vi "AddObject.vi"(6 "donating?":bool=TRUE, 8 "error in (no error)":errorcluster, 9 "Ancestor":string, 10 "driver":refnum<class "ViPER.lvclass">, 11 "reference in":refnum<class "ViPER.lvclass">) -> (0 "error out":errorcluster, 3 "reference out":refnum<class "ViPER.lvclass">)   [LabVIEW 2022 SP3, in "ViPER.lvlib" / "ViPER.lvclass"]
doc: "### BSD License (http://www.opensource.org/licenses/bsd-license.php) Begin ###\n\nCopyright (c) 2018 Kurt Friday www.medulla.net\n\nAll rights reserved.\n\nRedistribution and use in source and binary forms, with or without\nmodification, are permitted provided that the following conditions are met:\n\n * Redistributions of source code must retain the above copyright\n notice, this list of conditions and the following disclaimer.\n\n * Redistributions in binary form must reproduce the above copyright\n notice, this list of conditions and the following disclaimer in the\n documentation and/or other materials provided with the distribution.\n\n * Neither the name of the <organization> nor the\n names of its contributors may be used to endorse or promote products\n derived from this software without specific prior written permission.\n\nTHIS SOFTWARE IS PROVIDED BY THE COPYRIGHT HOLDERS AND CONTRIBUTORS \"AS IS\" AND\nANY EXPRESS OR IMPLIED WARRANTIES, INCLUDING, BUT NOT LIMITED TO, THE IMPLIED\nWARRANTIES OF MERCHANTABILITY AND FITNESS FOR A PARTICULAR PURPOSE ARE\nDISCLAIMED. IN NO EVENT SHALL <COPYRIGHT HOLDER> BE LIABLE FOR ANY\nDIRECT, INDIRECT, INCIDENTAL, SPECIAL, EXEMPLARY, OR CONSEQUENTIAL DAMAGES\n(INCLUDING, BUT NOT LIMITED TO, PROCUREMENT OF SUBSTITUTE GOODS OR SERVICES;\nLOSS OF USE, DATA, OR PROFITS; OR BUSINESS INTERRUPTION) HOWEVER CAUSED AND\nON ANY THEORY OF LIABILITY, WHETHER IN CONTRACT, STRICT LIABILITY, OR TORT\n(INCLUDING NEGLIGENCE OR OTHERWISE) ARISING IN ANY WAY OUT OF THE USE OF THIS\nSOFTWARE, EVEN IF ADVISED OF THE POSSIBILITY OF SUCH DAMAGE."
uses:
  ViPER.lvclass
  ObjectLayers.ctl
panel:
  # "### BSD License (http://www.opensource.org/licenses/bsd-license.php) Begin ###\n\nCopyright (c) 2018  Kurt Friday www.medulla.net\n\nAll rights reserved.\n\nRedistribution and use in source and binary forms, with or without\nmodification, are permitted provided that the following conditions are met:\n\n    * Redistributions of source code must retain the above copyright\n      notice, this list of conditions and the following disclaimer.\n\n    * Redistributions in binary form must reproduce the above copyright\n      notice, this list of conditions and the following disclaimer in the\n      documentation and/or other materials provided with the distribution.\n\n    * Neither the name of the <organization> nor the\n      names of its contributors may be used to endorse or promote products\n      derived from this software without specific prior written permission.\n\nTHIS SOFTWARE IS PROVIDED BY THE COPYRIGHT HOLDERS AND CONTRIBUTORS \"AS IS\" AND\nANY EXPRESS OR IMPLIED WARRANTIES, INCLUDING, BUT NOT LIMITED TO, THE IMPLIED\nWARRANTIES OF MERCHANTABILITY AND FITNESS FOR A PARTICULAR PURPOSE ARE\nDISCLAIMED. IN NO EVENT SHALL <COPYRIGHT HOLDER> BE LIABLE FOR ANY\nDIRECT, INDIRECT, INCIDENTAL, SPECIAL, EXEMPLARY, OR CONSEQUENTIAL DAMAGES\n(INCLUDING, BUT NOT LIMITED TO, PROCUREMENT OF SUBSTITUTE GOODS OR SERVICES;\nLOSS OF USE, DATA, OR PROFITS; OR BUSINESS INTERRUPTION) HOWEVER CAUSED AND\nON ANY THEORY OF LIABILITY, WHETHER IN CONTRACT, STRICT LIABILITY, OR TORT\n(INCLUDING NEGLIGENCE OR OTHERWISE) ARISING IN ANY WAY OUT OF THE USE OF THIS\nSOFTWARE, EVEN IF ADVISED OF THE POSSIBILITY OF SUCH DAMAGE."
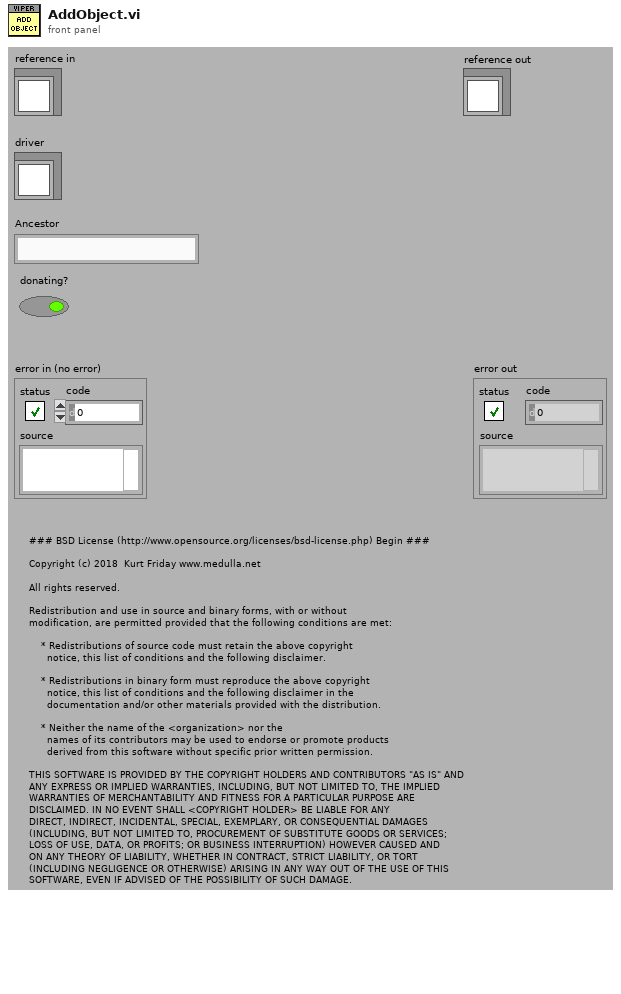
[diagram p1: front panel]
types:
  T1 = typedef "ViPER.lvlib/ViPER.lvclass/ObjectLayers.ctl" = cluster{"Ancestor":string, "Objects":refnum<class "ViPER.lvclass">[], "Object_Names":string[], "Owned":bool[]}
  T2 = typedef "ViPER.lvlib/ViPER.lvclass/ObjectAttributes.ctl" = cluster{"Object":T3, "Ancestors":T1[], "Config":T5, "Init_OK":bool, "Hierachy":string[], "PPL?":bool[], "SFP_Open":bool[], "Config_SFP_Open":bool[], "SoftFP_event":refnum<user-event>[], "ConfigFP_event":refnum<user-event>[], "SoftFP_Shutdown_Notifier":refnum<notifier>[], "ConfigFP_Shutdown_Notifier":refnum<notifier>[]}
  T3 = typedef "ViPER.lvlib/ViPER.lvclass/ObjectDefinition.ctl" = cluster{"Name":string, "Ancestors":T4[]}
  T4 = typedef "ViPER.lvlib/ViPER.lvclass/Ancestor.ctl" = cluster{"Class":string, "Config":string, "Objects":string[]}
  T5 = typedef "ViPER.lvlib/ViPER.lvclass/Config.ctl" = cluster{"default":string}
  T6 = typedef "ViPER.lvlib/ViPER.lvclass/Details.ctl" = cluster{"Name":string, "Class":string}
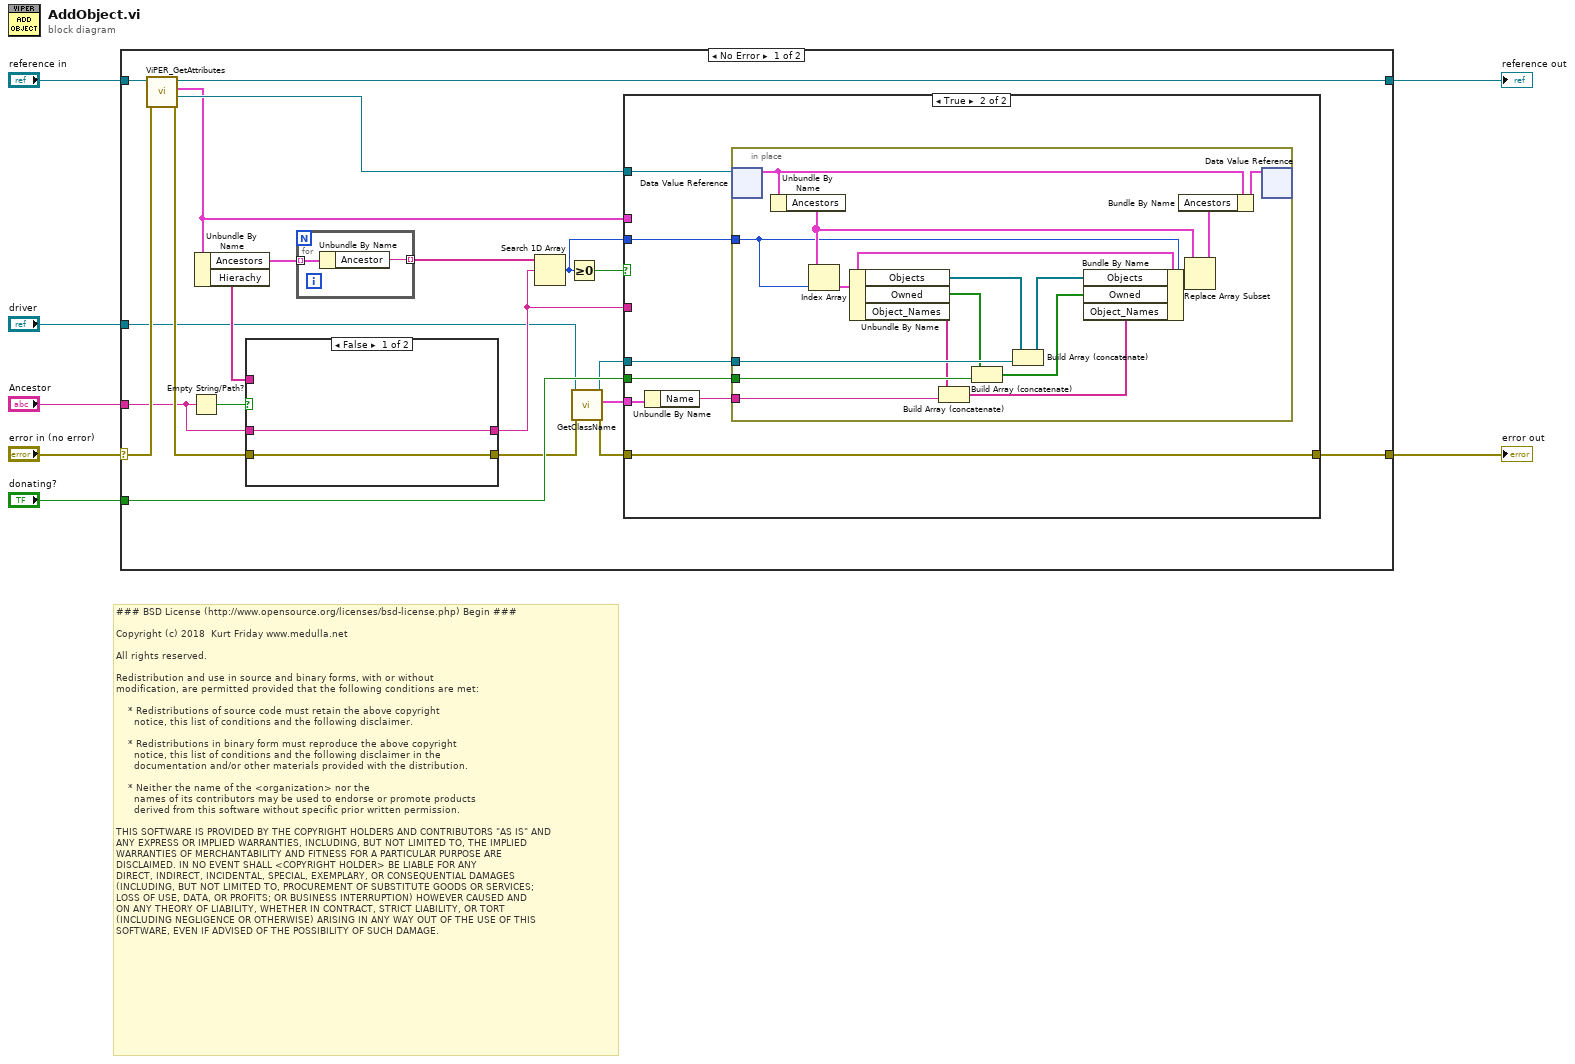
[diagram p0: block diagram]
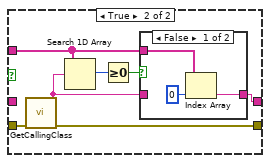
[diagram p2: hidden frame]
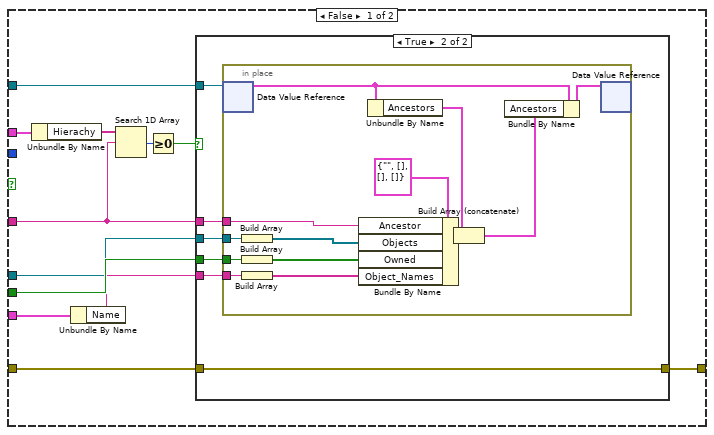
[diagram p4: hidden frame]
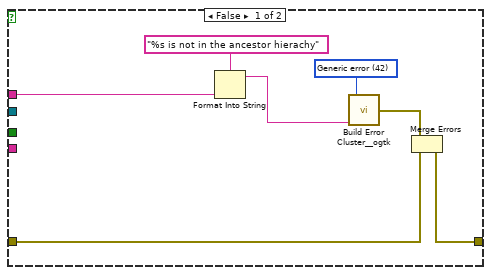
[diagram p5: hidden frame]
diagram:
  # "### BSD License (http://www.opensource.org/licenses/bsd-license.php) Begin ###\n\nCopyright (c) 2018  Kurt Friday www.medulla.net\n\nAll rights reserved.\n\nRedistribution and use in source and binary forms, with or without\nmodification, are permitted provided that the following conditions are met:\n\n    * Redistributions of source code must retain the above copyright\n      notice, this list of conditions and the following disclaimer.\n\n    * Redistributions in binary form must reproduce the above copyright\n      notice, this list of conditions and the following disclaimer in the\n      documentation and/or other materials provided with the distribution.\n\n    * Neither the name of the <organization> nor the\n      names of its contributors may be used to endorse or promote products\n      derived from this software without specific prior written permission.\n\nTHIS SOFTWARE IS PROVIDED BY THE COPYRIGHT HOLDERS AND CONTRIBUTORS \"AS IS\" AND\nANY EXPRESS OR IMPLIED WARRANTIES, INCLUDING, BUT NOT LIMITED TO, THE IMPLIED\nWARRANTIES OF MERCHANTABILITY AND FITNESS FOR A PARTICULAR PURPOSE ARE\nDISCLAIMED. IN NO EVENT SHALL <COPYRIGHT HOLDER> BE LIABLE FOR ANY\nDIRECT, INDIRECT, INCIDENTAL, SPECIAL, EXEMPLARY, OR CONSEQUENTIAL DAMAGES\n(INCLUDING, BUT NOT LIMITED TO, PROCUREMENT OF SUBSTITUTE GOODS OR SERVICES;\nLOSS OF USE, DATA, OR PROFITS; OR BUSINESS INTERRUPTION) HOWEVER CAUSED AND\nON ANY THEORY OF LIABILITY, WHETHER IN CONTRACT, STRICT LIABILITY, OR TORT\n(INCLUDING NEGLIGENCE OR OTHERWISE) ARISING IN ANY WAY OUT OF THE USE OF THIS\nSOFTWARE, EVEN IF ADVISED OF THE POSSIBILITY OF SUCH DAMAGE."
  n1 = case shown="No Error" "error in (no error)" {
    selector: "error in (no error)" -> [w26 w106]
    tunnel: [w22 w106] -> w6
    tunnel: [w27 w105] -> w4
    tunnel: "reference in" -> [w28 w105]
    tunnel: "driver" -> [w12 _]
    tunnel: "donating?" -> [w17 _]
    tunnel: "Ancestor" -> [w13 _]
    frame No Error {
      n2 = call "ViPER_GetAttributes.vi"("error in (no error)"=w26, "reference in"=w28) -> ("error out"=w19:errorcluster, "DataRef"=w20:refnum<data-value>, "Data"=w15:T2, "reference out"=w27:refnum<class "ViPER.lvclass">)  [unwired: 6 in]
      n3 = Empty String/Path?(string/path=w13) -> (empty?=w16:bool)
      n4 = Unbundle By Name(w15) -> ("Ancestors"=w25:T1[], "Hierachy"=w14:string[])
      n5 = case shown="False" w16 {
        tunnel: w19 -> [w30 w37]
        tunnel: [w30 w36] -> w9
        tunnel: [w29 w32] -> w18
        tunnel: w13 -> [w29 _]
        tunnel: w14 -> [_ w33]
        frame False {
        }
        frame True {
          n6 = call "GetCallingClass.vi"("error in (no error)"=w37) -> ("error out"=w36:errorcluster, "calling class"=w31:string)  [unwired: 9 in]
          n7 = Search 1D Array(1D array=w33, element=w31) -> (index of element=w35:i32)  [unwired: 1 in]
          n8 = Greater Or Equal To 0?(x=w35) -> (x >= 0?=w34:bool)
          n9 = case shown="False" w34 {
            tunnel: w33 -> [w40 _]
            tunnel: [w38 w41] -> w32
            tunnel: w31 -> [_ w41]
            frame False {
              n10 = Index Array(array=w40, index=0) -> (element=w38:string)
            }
            frame True {
            }
          }
        }
      }
      n11 = for {
        tunnel: w25 -> [w104] mode=indexing
        tunnel: [w103] -> w24 mode=indexing
        n12 = Unbundle By Name(w104) -> ("Ancestor"=w103:string)
      }
      n13 = Search 1D Array(1D array=w24, element=w18) -> (index of element=w21:i32)  [unwired: 1 in]
      n14 = Greater Or Equal To 0?(x=w21) -> (x >= 0?=w23:bool)
      n15 = call "GetClassName.vi"("error in (no error)"=w9, "reference in"=w12) -> ("error out"=w10:errorcluster, "Details"=w8:T6, "reference out"=w11:refnum<class "ViPER.lvclass">)  [unwired: 7 in]
      n16 = case shown="True" w23 {
        tunnel: w10 -> [w43 w86]
        tunnel: [w47 w86] -> w22
        tunnel: w21 -> [_ w84]
        tunnel: w20 -> [w53 w85]
        tunnel: w11 -> [w44 w83]
        tunnel: w18 -> [w50 _]
        tunnel: w17 -> [w46 w82]
        tunnel: w15 -> [w52 _]
        tunnel: w8 -> [w42 w81]
        frame False {
          n17 = Unbundle By Name(w52) -> ("Hierachy"=w51:string[])
          n18 = Unbundle By Name(w42) -> ("Name"=w45:string)
          n19 = Search 1D Array(1D array=w51, element=w50) -> (index of element=w49:i32)  [unwired: 1 in]
          n20 = Greater Or Equal To 0?(x=w49) -> (x >= 0?=w48:bool)
          n21 = case shown="True" w48 {
            tunnel: w53 -> [_ w66]
            tunnel: w44 -> [_ w65]
            tunnel: w50 -> [w56 w64]
            tunnel: w46 -> [_ w63]
            tunnel: w43 -> [w60 w62]
            tunnel: [w58 w62] -> w47
            tunnel: w45 -> [_ w61]
            frame False {
              w57 = 42 items=["No error", "Argument error", "Memory is full", "Out of zone", "End of file", "File already open", "Generic file I/O error", "File not found", "File permission error", "Disk is full", "Duplicate path", "Too many files open", "System feature not enabled", "Resource file not found", "Cannot add resource", "Resource not found", "Image not found", "Image memory error", "Pen does not exist", "Config type invalid", "Config token not found", "Config parse error", "Config memory error", "Bad external code format", "Bad external code offset", "External code not present", "Null window", "Destroy window error", "Null menu", "Print aborted", "Bad print record", "Print driver error", "Windows error during printing", "Memory error during printing", "Print dialog error", "Generic print error", "Invalid device refnum", "Device not found", "Device parameter error", "Device unit error", "Cannot open device", "Device call aborted", "Generic error", "Cancelled by user", "Object ID too low", "Object ID too high", "Object not in heap", "Unknown heap", "Unknown object (invalid DefProc)", "Unknown object (DefProc not in table)", "Message out of range", "Invalid (null) method", "Unknown message", "Manager call not supported", "Bad address", "Network operation in progress", "Network operation timed out", "Connection is busy", "Network attribute not supported", "Network error", "Address in use", "System out of memory", "Connection aborted", "Connection refused", "Not connected", "Already connected", "Connection closed", "Initialization error (interapplication manager)", "Bad occurrence", "Wait on unbound occurrence handler", "Occurrence queue overflow", "Datalog type conflict", "Unused", "Unrecognized type (interapplication manager)", "Memory corrupt", "Failed to make temporary DLL", "Old CIN version", "Drag socket not found", "Failed to load drop-object", "Failed to register OLE object", "Failed to release OLE object", "Format specifier type mismatch", "Unknown format specifier", "Too few format specifiers", "Too many format specifiers", "Scan failed", "Newer CIN version", "Error converting to variant", "Runtime menu error", "Password tampered", "Variant attribute not found", "Incompatible variant data type", "Event data is not available", "Event Store is not present", "Occurrence is not found", "Event Queue is not created", "Event info is not available", "Refnum passed is NULL", "Error retrieving Class GUID", "Error retrieving CoClass GUID", "Error retrieving TypeLib GUID.", "Bad built application magic bytes.", "Specific driver is different from the specific driver associated with the Logical Name.", "There is no session opened to the class driver.", "Max Error", "MAX - Error with config objects", "MAX - Error loading configuration", "MAX - Group not supported"]
              n22 = Format Into String(format string="%s is not in the ancestor hierachy", w56) -> (resulting string=w54:string)  [unwired: 2 in, 1 out]
              n23 = call <userlib>:"Build Error Cluster__ogtk.vi"("String to Prepend to source (\"\")"=w54, "code"=w57) -> ("error out"=w59:errorcluster)
              n24 = Merge Errors(w59, w60) -> (w58:errorcluster)
            }
            frame True {
              n25 = in-place {
                in-place-border: w65 -> [w77]
                in-place-border: w64 -> [w71]
                in-place-border: w63 -> [w70]
                in-place-border: w61 -> [w68]
                n26 = in-place-dvr #1(w66) -> (w78:T2)  [unwired: 1 out]
                n27 = Build Array(w77) -> (w73:refnum<class "ViPER.lvclass">[])
                n28 = Build Array(w70) -> (w69:bool[])
                n29 = Build Array(w68) -> (w67:string[])
                n30 = Bundle By Name(cluster=T1 {"Ancestor"="", "Objects"=[], "Object_Names"=[], "Owned"=[]} ("Layer"), "Ancestor"=w71, "Objects"=w73, "Owned"=w69, "Object_Names"=w67) -> (w72:T1)
                n31 = Unbundle By Name(w78) -> ("Ancestors"=w76:T1[])
                n32 = Build Array (concatenate)(w76, w72) -> (w75:T1[])
                n33 = Bundle By Name(cluster=w78, "Ancestors"=w75) -> (w79:T2)
                n34 = in-place-dvr #1(w79) -> ()  [unwired: 2 out]
              }
            }
          }
        }
        frame True {
          n35 = Unbundle By Name(w81) -> ("Name"=w80:string)
          n36 = in-place {
            in-place-border: w84 -> [w99]
            in-place-border: w83 -> [w94]
            in-place-border: w82 -> [w90]
            in-place-border: w80 -> [w87]
            n37 = in-place-dvr #2(w85) -> (w101:T2)  [unwired: 1 out]
            n38 = Unbundle By Name(w101) -> ("Ancestors"=w100:T1[])
            n39 = Index Array(array=w100, index=w99) -> (element=w97:T1)
            n40 = Unbundle By Name(w97) -> ("Objects"=w98:refnum<class "ViPER.lvclass">[], "Owned"=w92:bool[], "Object_Names"=w89:string[])
            n41 = Build Array (concatenate)(w89, w87) -> (w88:string[])
            n42 = Build Array (concatenate)(w92, w90) -> (w91:bool[])
            n43 = Build Array (concatenate)(w98, w94) -> (w95:refnum<class "ViPER.lvclass">[])
            n44 = Bundle By Name(cluster=w97, "Objects"=w95, "Owned"=w91, "Object_Names"=w88) -> (w96:T1)
            n45 = Replace Array Subset(array=w100, new element=w96, index=w99) -> (w93:T1[])
            n46 = Bundle By Name(cluster=w101, "Ancestors"=w93) -> (w102:T2)
            n47 = in-place-dvr #2(w102) -> ()  [unwired: 2 out]
          }
        }
      }
    }
    frame Error {
    }
  }
  "error out" <- w6
  "reference out" <- w4
